vi "Teleop.vi"(10 "Match Info":T2={"Autonomous Elapsed Seconds"=0.0, "TeleOp Elapsed Seconds"=0.0, "Disabled Elapsed Seconds"=0.0, "Visited Autonomous"=FALSE, "Visited TeleOp"=FALSE, "Visited Disabled"=FALSE, "Autonomous Settings"={"Autonomous Style"=enum."Independent", "VI Refnum"=refnum}}, 11 "Call Context":T3) -> ()   [LabVIEW 2020]
doc: "This VI is called for each TeleOp packet received from the DS where the robot is not disabled. It is often used to read from the joysticks and update I/O or to update setpoints for timed control loops. It should complete and return within 20 milliseconds or it may miss DS packets."
uses:
  <vilib>/Rock Robotics/WPI/DriverStation/WPI_DriverStationDerivedRobotMode.ctl
  <vilib>/Rock Robotics/WPI/DriverStation/WPI_DriverStationMatch Info.ctl
  <vilib>/Rock Robotics/WPI/ThirdParty/Phoenix-LabVIEW/Motor Controller/Controls/CTRE_Phoenix_MotorControl_ControlMode.ctl
  <vilib>/Rock Robotics/WPI/ThirdParty/Phoenix-LabVIEW/CANCoder/Get/CTRE_Phoenix_CANcoder_GetSensorData.vi
  <vilib>/Rock Robotics/WPI/ThirdParty/Phoenix-LabVIEW/Pigeon IMU/CTRE_PigeonIMU_GetYPR.vi
panel:
  in  "FR PID gains":T1={"proportional gain (Kc)"=0.01, "integral time (Ti, min)"=0.0, "derivative time (Td, min)"=0.0} {"derivative time (Td, min)" format="%.3f"; "integral time (Ti, min)" format="%.3f"; "proportional gain (Kc)" format="%.6f"}
  in  "FL PID gains":T1={"proportional gain (Kc)"=0.01, "integral time (Ti, min)"=0.0, "derivative time (Td, min)"=0.0} {"derivative time (Td, min)" format="%.3f"; "integral time (Ti, min)" format="%.3f"; "proportional gain (Kc)" format="%.6f"}
  in  "BR PID gains":T1={"proportional gain (Kc)"=0.01, "integral time (Ti, min)"=0.0, "derivative time (Td, min)"=0.0} {"derivative time (Td, min)" format="%.3f"; "integral time (Ti, min)" format="%.3f"; "proportional gain (Kc)" format="%.6f"}
  in  "BL PID gains":T1={"proportional gain (Kc)"=0.01, "integral time (Ti, min)"=0.0, "derivative time (Td, min)"=0.0} {"derivative time (Td, min)" format="%.3f"; "integral time (Ti, min)" format="%.3f"; "proportional gain (Kc)" format="%.6f"}
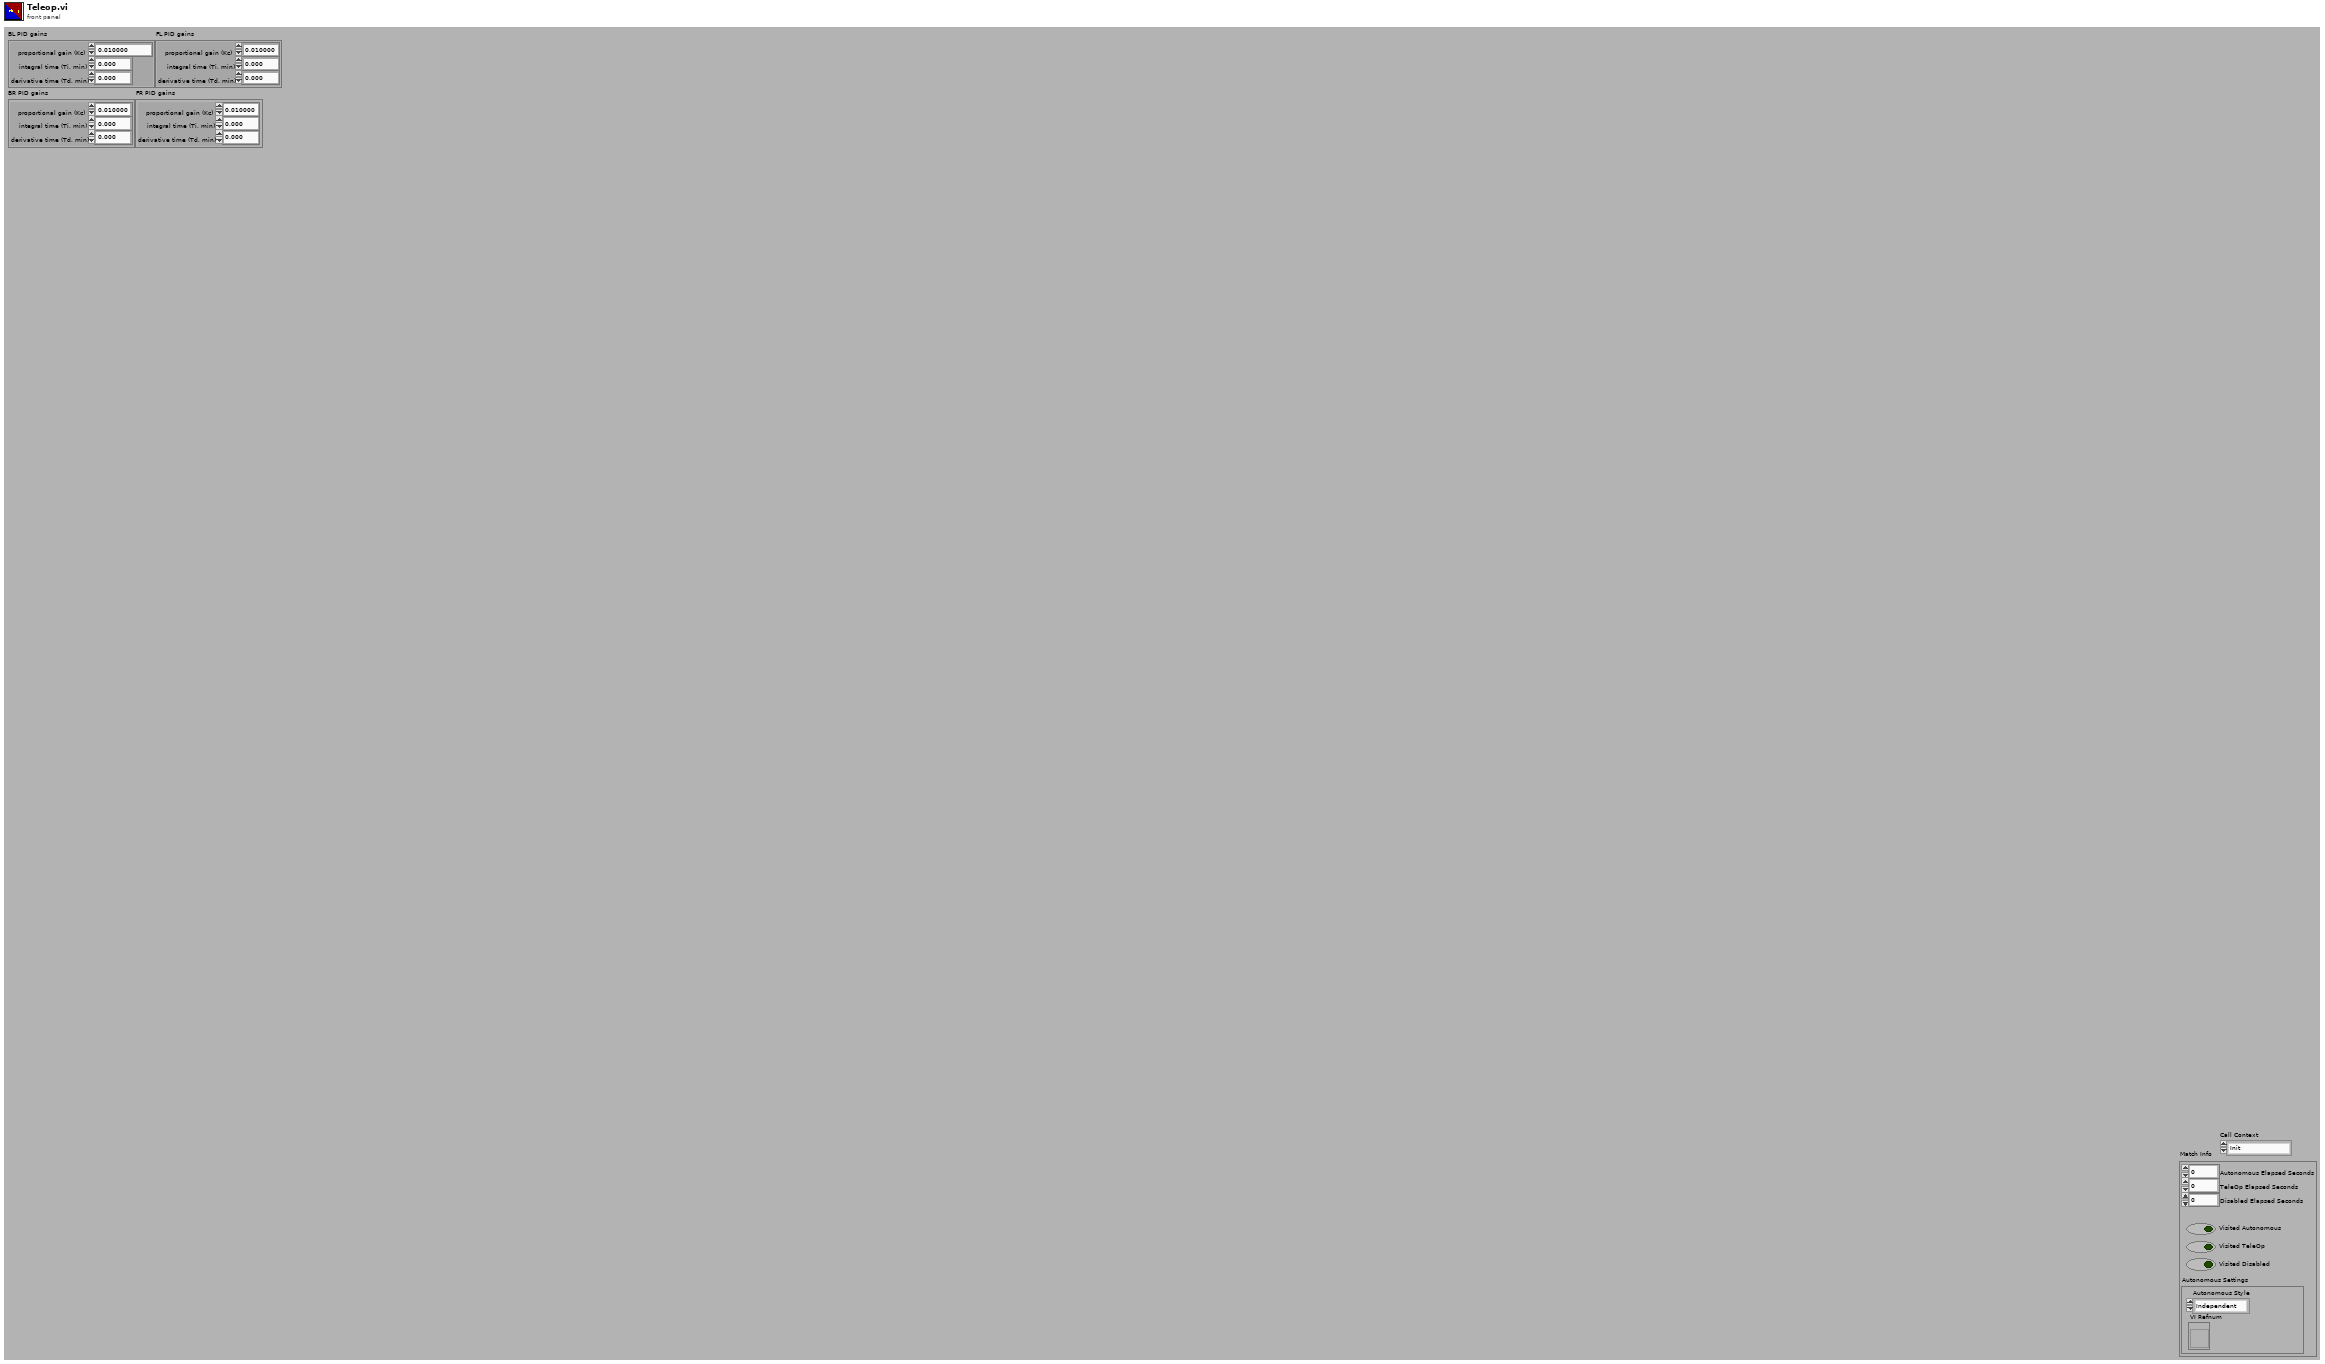
[diagram p1: front panel]
types:
  T1 = cluster{"proportional gain (Kc)":dbl, "integral time (Ti, min)":dbl, "derivative time (Td, min)":dbl}
  T2 = typedef "WPI_DriverStationMatch Info.ctl" = cluster{"Autonomous Elapsed Seconds":dbl, "TeleOp Elapsed Seconds":dbl, "Disabled Elapsed Seconds":dbl, "Visited Autonomous":bool, "Visited TeleOp":bool, "Visited Disabled":bool, "Autonomous Settings":cluster{"Autonomous Style":enum16{"Iterative", "Independent"}, "VI Refnum":refnum<vi>}}
  T3 = typedef "WPI_DriverStationDerivedRobotMode.ctl" = enum16{"Init", "Execute", "Stop"}
  T4 = typedef "CTRE_Phoenix_MotorControl_ControlMode.ctl" = u16
  T5 = cluster{"A":bool, "B":bool, "X":bool, "Y":bool, "Left Bumper":bool, "Right Bumper":bool, "View Button":bool, "Menu Button":bool, "Left Joystick Press":bool, "Right Joystick Press":bool, "Left Thumbpad X Axis":dbl, "Left Thumbpad Y Axis":dbl, "Left Trigger":dbl, "Right Trigger":dbl, "Right Thumbpad X Axis":dbl, "Right Thumbpad Y Axis":dbl, "Driver - Trigger":bool, "Driver - Middle Thumb":bool, "Driver - Left Thumb":bool, "Driver - Right Thumb":bool, "Driver - Left Top Left ":bool, "Driver - Left Top Middle":bool, "Driver - Left Top Right":bool, "Driver - Left Bottom Right":bool, "Driver - Left Bottom Middle":bool, "Driver - Left Bottom Left":bool, "Driver - Right Top Right":bool, "Driver - Right Top Middle":bool, "Driver - Right Top Left":bool, "Driver - Right Bottom Left":bool, "Driver - Right Bottom Middle":bool, "Driver - Right Bottom Right":bool, "Driver - X Axis":dbl, "Driver - Y Axis":dbl, "Driver - Z Axis":dbl}
  T6 = typedef "CTRE_PigeonIMU_DeviceRef.ctl" = cluster{"DeviceStatus":errorcluster, "Device Number":u8, "Type":T7, "Device ID":u32, "Handle":u64, "UsageFrame":u32, "Library Path":path}
  T7 = typedef "CTRE_PigeonIMU_ConnectionType.ctl" = u32
  T8 = typedef "CTRE_Phoenix_CANcoder_DeviceRef.ctl" = cluster{"DeviceStatus":errorcluster, "Device Number":u8, "Handle":u64, "UsageFrame":u32, "Library Path":path}
  T9 = typedef "WPI_MotorControlDeviceRef.ctl" = cluster{"DeviceStatus":errorcluster, "Type":T10, "PWM":cluster{"PWM Channel":T11, "DeadBand":T12}, "CAN":cluster{"Device Number":u8, "SetOutput VI Ref":variant, "GetOutput VI Ref":variant, "Enable VI Ref":variant, "Disable VI Ref":variant, "Data":variant}, "Invert":bool, "DIO PWM":cluster{"PWM \"Enable\" Channel":T11, "DIOChannel":T13, "PWM Rate":dbl}}
  T10 = typedef "WPI_MotorControlType.ctl" = enum16{"PWM", "CAN", "DIO PWM"}
  T11 = typedef "FPGA_DIOPWMChannel.ctl" = enum8{"PWM 0", "PWM 1", "PWM 2", "PWM 3", "PWM 4", "PWM 5", "PWM 6", "PWM 7", "PWM 8", "PWM 9", "PWM MXP 0", "PWM MXP 1", "PWM MXP 2", "PWM MXP 3", "PWM MXP 4", "PWM MXP 5", "PWM MXP 6", "PWM MXP 7", "PWM MXP 8", "PWM MXP 9", "Invalid"}
  T12 = typedef "WPI_PWMDeadband.ctl" = cluster{"Name":string, "maxPositivePwm":i32, "minPositivePwm":i32, "centerPwm":i32, "maxNegativePwm":i32, "minNegativePwm":i32, "angularRange":u16}
  T13 = typedef "FPGA_DIOChannel.ctl" = enum8{"DIO 0", "DIO 1", "DIO 2", "DIO 3", "DIO 4", "DIO 5", "DIO 6", "DIO 7", "DIO 8", "DIO 9", "DIO MXP 0", "DIO MXP 1", "DIO MXP 2", "DIO MXP 3", "DIO MXP 4", "DIO MXP 5", "DIO MXP 6", "DIO MXP 7", "DIO MXP 8", "DIO MXP 9", "DIO MXP 10", "DIO MXP 11", "DIO MXP 12", "DIO MXP 13", "DIO MXP 14", "DIO MXP 15", "SPI Port CS1", "SPI Port CS2", "SPI Port CS3", "SPI Port MISO", "SPI Port MOSI", "Invalid"}
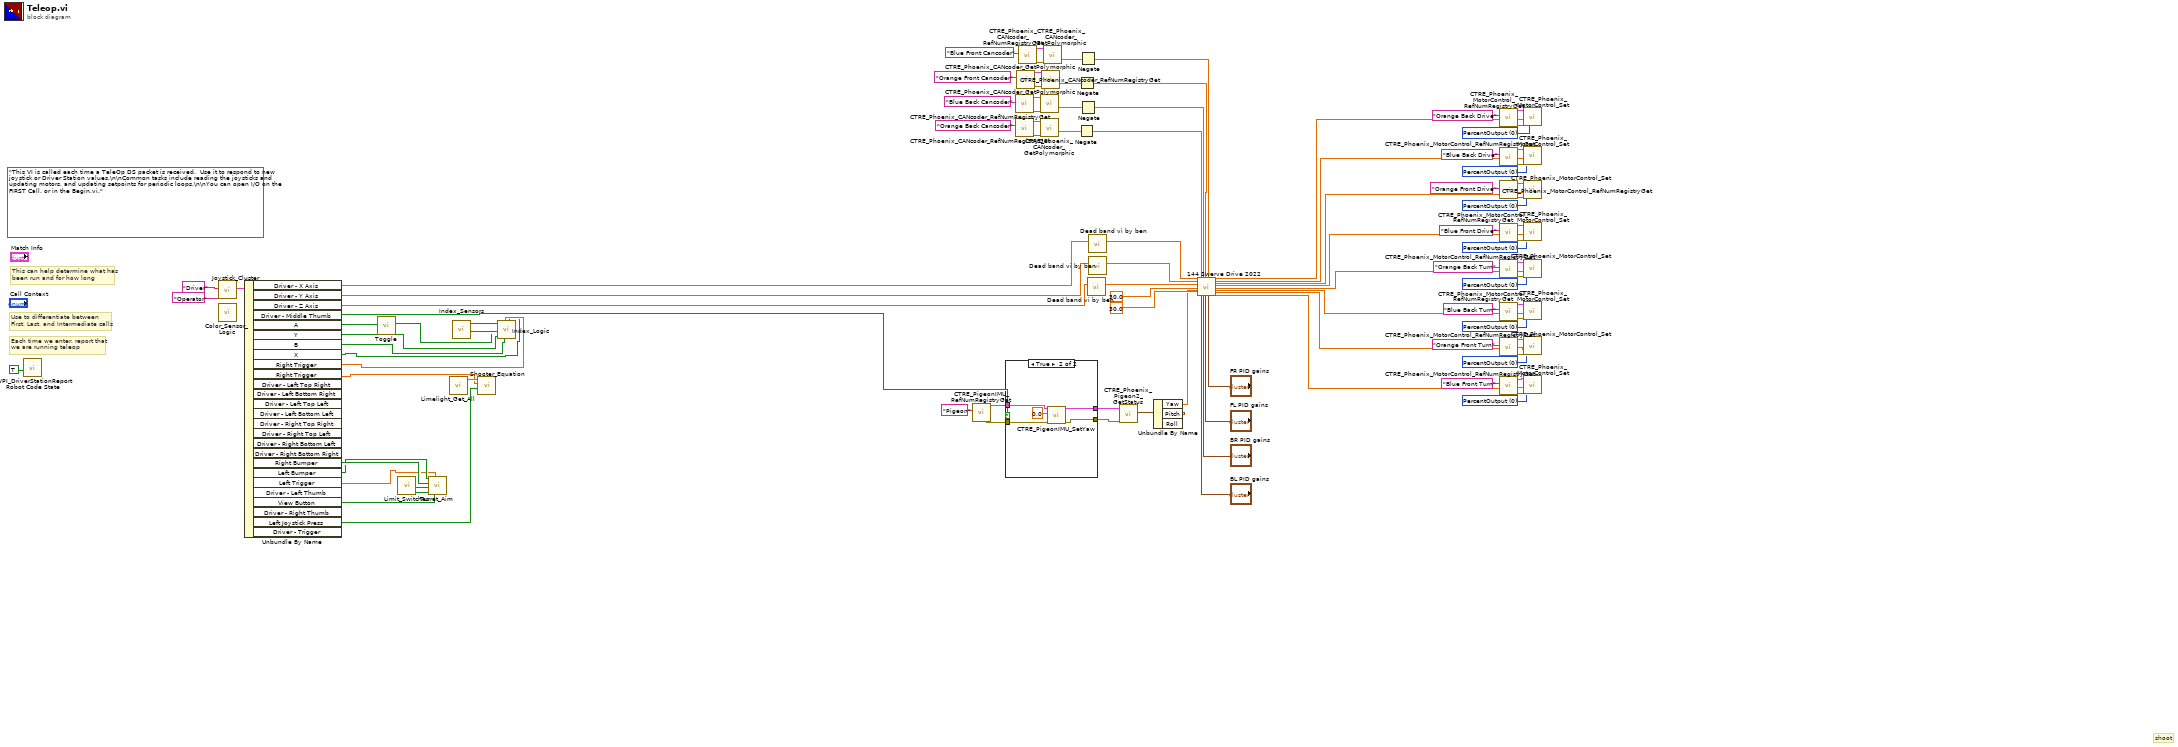
[diagram p0: block diagram]
diagram:
  w14 = T4 0 items=["PercentOutput"=0, "Position"=1, "Velocity"=2, "Current"=3, "Follower"=5, "MotionProfile"=6, "MotionMagic"=7, "MotionProfileArc"=10, "Disabled"=15] ("Control Mode")
  w18 = T4 0 items=["PercentOutput"=0, "Position"=1, "Velocity"=2, "Current"=3, "Follower"=5, "MotionProfile"=6, "MotionMagic"=7, "MotionProfileArc"=10, "Disabled"=15] ("Control Mode")
  w21 = T4 0 items=["PercentOutput"=0, "Position"=1, "Velocity"=2, "Current"=3, "Follower"=5, "MotionProfile"=6, "MotionMagic"=7, "MotionProfileArc"=10, "Disabled"=15] ("Control Mode")
  w25 = T4 0 items=["PercentOutput"=0, "Position"=1, "Velocity"=2, "Current"=3, "Follower"=5, "MotionProfile"=6, "MotionMagic"=7, "MotionProfileArc"=10, "Disabled"=15] ("Control Mode")
  w53 = T4 0 items=["PercentOutput"=0, "Position"=1, "Velocity"=2, "Current"=3, "Follower"=5, "MotionProfile"=6, "MotionMagic"=7, "MotionProfileArc"=10, "Disabled"=15] ("Control Mode")
  w57 = T4 0 items=["PercentOutput"=0, "Position"=1, "Velocity"=2, "Current"=3, "Follower"=5, "MotionProfile"=6, "MotionMagic"=7, "MotionProfileArc"=10, "Disabled"=15] ("Control Mode")
  w60 = T4 0 items=["PercentOutput"=0, "Position"=1, "Velocity"=2, "Current"=3, "Follower"=5, "MotionProfile"=6, "MotionMagic"=7, "MotionProfileArc"=10, "Disabled"=15] ("Control Mode")
  w4 = T4 0 items=["PercentOutput"=0, "Position"=1, "Velocity"=2, "Current"=3, "Follower"=5, "MotionProfile"=6, "MotionMagic"=7, "MotionProfileArc"=10, "Disabled"=15] ("Control Mode")
  (unwired) "This VI is called each time a TeleOp DS packet is received.  Use it to respond to new joystick or Driver Station values.\n\nCommon tasks include reading the joysticks and updating motors, and updating setpoints for periodic loops.\n\nYou can open I/O on the FIRST Call, or in the Begin.vi."
  # "shoot"
  # "Each time we enter, report that\nwe are running teleop"
  # "Use to differentiate between\nFirst, Last, and Intermediate calls"
  # "This can help determine what has\nbeen run and for how long"
  n1 = call <vilib>:"WPI_DriverStationReport Robot Code State.vi"("TeleOp"=TRUE ("Autonomous")) -> ()  [unwired: 10 in, 1 out]
  n2 = call "Joystick_Cluster.vi"("Xbox"="Operator", "Thrustmaster"="Driver") -> ("Joystick Output"=w98:T5)  [unwired: 9 in]
  n3 = call "Color_Sensor_Logic.vi"() -> ()  [unwired: 12 in]
  n4 = Unbundle By Name(w98) -> ("Driver - X Axis"=w36:dbl, "Driver - Y Axis"=w35:dbl, "Driver - Z Axis"=w34:dbl, "Driver - Middle Thumb"=w41:bool, "A"=w92:bool, "Y"=w95:bool, "B"=w94:bool, "X"=w1:bool, "Right Trigger"=w93:dbl, "Right Trigger"=w89:dbl, "Right Bumper"=w86:bool, "Left Bumper"=w85:bool, "Left Trigger"=w84:dbl, "View Button"=w83:bool, "Left Joystick Press"=w2:bool)  [unwired: 11 out]
  n5 = call "Toggle.vi"("Boolean"=w92) -> ("Boolean Out"=w91:bool)
  n6 = call "Limit_Switches.vi"() -> ("Blue Limit Pressed"=w87:bool, "Orange Limit Pressed"=w88:bool)  [unwired: 10 in]
  n7 = call "Turret_Aim.vi"("View Button"=w83, "Left Trigger"=w84, "Orange Limit Pressed"=w88, "Blue Limit Pressed"=w87, "Right Bumper"=w86, "Left Bumper"=w85) -> ()  [unwired: 6 in]
  n8 = call "Limelight_Get_All.vi"() -> ("Ty"=w90:dbl)  [unwired: 10 in, 1 out]
  n9 = call "Index_Sensors.vi"() -> ("Intake Pressed"=w97:bool, "Elevate Pressed"=w96:bool)  [unwired: 9 in, 1 out]
  n10 = call "Shooter_Equation.vi"("Left Bumper"=w2, "Right Trigger"=w89, "Ty"=w90) -> ()  [unwired: 9 in]
  n11 = call "Index_Logic.vi"("Intake Pressed"=w97, "X"=w1, "B"=w94, "Right Trigger"=w93, "Y"=w95, "A"=w91, "Elevate Pressed"=w96) -> ()  [unwired: 5 in]
  n12 = call <vilib>:"CTRE_PigeonIMU_RefNumRegistryGet.vi"("refnum name"="Pigeon") -> ("error out"=w50:errorcluster, "PigeonIMUDevRef"=w51:T6)  [unwired: 9 in]
  n13 = case shown="True" w41 {
    tunnel: w51 -> [w103 w107]
    tunnel: w50 -> [w102 w106]
    tunnel: [w102 w105] -> w49
    tunnel: [w103 w104] -> w48
    frame False {
    }
    frame True {
      n14 = call <vilib>:"CTRE_PigeonIMU_SetYaw.vi"("error in (no error)"=w106, "Value"=0.0, "PigeonIMUDevRef"=w107) -> ("error out"=w105:errorcluster, "PigeonIMUDevRef"=w104:T6)  [unwired: 7 in]
    }
  }
  n15 = call <vilib>:"CTRE_Phoenix_CANcoder_RefNumRegistryGet.vi"("refnum name"="Blue Back Cancoder") -> ("error out"=w77:errorcluster, "CTRE_CANcoder_DeviceRef"=w78:T8)  [unwired: 9 in]
  n16 = call <vilib>:"CTRE_Phoenix_CANcoder_RefNumRegistryGet.vi"("refnum name"="Orange Back Cancoder") -> ("error out"=w79:errorcluster, "CTRE_CANcoder_DeviceRef"=w80:T8)  [unwired: 9 in]
  n17 = call <vilib>:"CTRE_Phoenix_CANcoder_RefNumRegistryGet.vi"("refnum name"="Orange Front Cancoder") -> ("error out"=w81:errorcluster, "CTRE_CANcoder_DeviceRef"=w82:T8)  [unwired: 9 in]
  n18 = call <vilib>:"CTRE_Phoenix_CANcoder_RefNumRegistryGet.vi"("refnum name"="Blue Front Cancoder") -> ("error out"=w75:errorcluster, "CTRE_CANcoder_DeviceRef"=w76:T8)  [unwired: 9 in]
  n19 = call-poly <vilib>:"CTRE_Phoenix_CANcoder_GetPolymorphic.vi"("CTRE_CANcoder_DeviceRef"=w78, "error in"=w77) -> ("Absolute Position"=w70:dbl)  [unwired: 9 in, 4 out]
  n20 = call-poly <vilib>:"CTRE_Phoenix_CANcoder_GetPolymorphic.vi"("CTRE_CANcoder_DeviceRef"=w80, "error in"=w79) -> ("Absolute Position"=w68:dbl)  [unwired: 9 in, 4 out]
  n21 = call-poly <vilib>:"CTRE_Phoenix_CANcoder_GetPolymorphic.vi"("CTRE_CANcoder_DeviceRef"=w82, "error in"=w81) -> ("Absolute Position"=w67:dbl)  [unwired: 9 in, 4 out]
  n22 = call-poly <vilib>:"CTRE_Phoenix_CANcoder_GetPolymorphic.vi"("CTRE_CANcoder_DeviceRef"=w76, "error in"=w75) -> ("Absolute Position"=w69:dbl)  [unwired: 9 in, 4 out]
  n23 = Negate(x=w68) -> (-x=w40:dbl)
  n24 = Negate(x=w67) -> (-x=w38:dbl)
  n25 = Negate(x=w69) -> (-x=w37:dbl)
  n26 = Negate(x=w70) -> (-x=w39:dbl)
  n27 = call "Dead band vi by ben.vi"("Numeric"=w34) -> ("Deadbanded Value"=w31:dbl)  [unwired: 10 in]
  n28 = call "Dead band vi by ben.vi"("Numeric"=w36) -> ("Deadbanded Value"=w33:dbl)  [unwired: 10 in]
  n29 = call "Dead band vi by ben.vi"("Numeric"=w35) -> ("Deadbanded Value"=w32:dbl)  [unwired: 10 in]
  n30 = call-poly <vilib>:"CTRE_Phoenix_Pigeon2_GetStatus.vi"("error in (no error)"=w49, "PigeonIMUDevRef"=w48) -> ("Yaw Pitch Roll"=w46:cluster{"Yaw":dbl, "Pitch":dbl, "Roll":dbl})  [unwired: 7 in, 2 out]
  n31 = Unbundle By Name(w46) -> ("Yaw"=w3:dbl)  [unwired: 2 out]
  n32 = call "144 Swerve Drive 2022.vi"("Joystick X"=w33, "Joystick Y"=w32, "Joystick Z"=w31, "Robot Length(in.)"=30.0, "Robot Width(in.)"=30.0, "Gyro"=w3, "BL_Steer_Encoder"=w40, "BL PID gains"="BL PID gains", "BR_Steer_Encoder"=w39, "BR PID gains"="BR PID gains", "FL_Steer_Encoder"=w38, "FL PID gains"="FL PID gains", "FR_Steer_Encoder"=w37, "FR PID gains"="FR PID gains") -> ("Throttle BL"=w12:dbl, "Throttle BR"=w11:dbl, "Throttle FL"=w10:dbl, "Throttle FR"=w9:dbl, "BL_STEER_MOTOR_OUTPUT"=w8:dbl, "BR_STEER_MOTOR_OUTPUT"=w7:dbl, "FL_STEER_MOTOR_OUTPUT"=w6:dbl, "FR_STEER_MOTOR_OUTPUT"=w5:dbl)  [unwired: 6 in]
  n33 = call <vilib>:"CTRE_Phoenix_MotorControl_RefNumRegistryGet.vi"("refnum name"="Orange Back Drive") -> ("error out"=w65:errorcluster, "PhoenixMotorControlDevRef"=w66:T9)  [unwired: 9 in]
  n34 = call <vilib>:"CTRE_Phoenix_MotorControl_RefNumRegistryGet.vi"("refnum name"="Blue Back Drive") -> ("error out"=w62:errorcluster, "PhoenixMotorControlDevRef"=w63:T9)  [unwired: 9 in]
  n35 = call <vilib>:"CTRE_Phoenix_MotorControl_RefNumRegistryGet.vi"("refnum name"="Orange Front Drive") -> ("error out"=w59:errorcluster, "PhoenixMotorControlDevRef"=w56:T9)  [unwired: 9 in]
  n36 = call <vilib>:"CTRE_Phoenix_MotorControl_RefNumRegistryGet.vi"("refnum name"="Blue Front Drive") -> ("error out"=w55:errorcluster, "PhoenixMotorControlDevRef"=w52:T9)  [unwired: 9 in]
  n37 = call <vilib>:"CTRE_Phoenix_MotorControl_RefNumRegistryGet.vi"("refnum name"="Orange Back Turn") -> ("error out"=w27:errorcluster, "PhoenixMotorControlDevRef"=w28:T9)  [unwired: 9 in]
  n38 = call <vilib>:"CTRE_Phoenix_MotorControl_RefNumRegistryGet.vi"("refnum name"="Blue Back Turn") -> ("error out"=w23:errorcluster, "PhoenixMotorControlDevRef"=w24:T9)  [unwired: 9 in]
  n39 = call <vilib>:"CTRE_Phoenix_MotorControl_RefNumRegistryGet.vi"("refnum name"="Orange Front Turn") -> ("error out"=w20:errorcluster, "PhoenixMotorControlDevRef"=w17:T9)  [unwired: 9 in]
  n40 = call <vilib>:"CTRE_Phoenix_MotorControl_RefNumRegistryGet.vi"("refnum name"="Blue Front Turn") -> ("error out"=w16:errorcluster, "PhoenixMotorControlDevRef"=w13:T9)  [unwired: 9 in]
  n41 = call <vilib>:"CTRE_Phoenix_MotorControl_Set.vi"("error in (no error)"=w65, "Output"=w12, "Control Mode"=w4, "PhoenixMotorControlDevRef"=w66) -> ()  [unwired: 6 in, 2 out]
  n42 = call <vilib>:"CTRE_Phoenix_MotorControl_Set.vi"("error in (no error)"=w62, "Output"=w11, "Control Mode"=w60, "PhoenixMotorControlDevRef"=w63) -> ()  [unwired: 6 in, 2 out]
  n43 = call <vilib>:"CTRE_Phoenix_MotorControl_Set.vi"("error in (no error)"=w59, "Output"=w10, "Control Mode"=w57, "PhoenixMotorControlDevRef"=w56) -> ()  [unwired: 6 in, 2 out]
  n44 = call <vilib>:"CTRE_Phoenix_MotorControl_Set.vi"("error in (no error)"=w55, "Output"=w9, "Control Mode"=w53, "PhoenixMotorControlDevRef"=w52) -> ()  [unwired: 6 in, 2 out]
  n45 = call <vilib>:"CTRE_Phoenix_MotorControl_Set.vi"("error in (no error)"=w27, "Output"=w8, "Control Mode"=w25, "PhoenixMotorControlDevRef"=w28) -> ()  [unwired: 6 in, 2 out]
  n46 = call <vilib>:"CTRE_Phoenix_MotorControl_Set.vi"("error in (no error)"=w23, "Output"=w7, "Control Mode"=w21, "PhoenixMotorControlDevRef"=w24) -> ()  [unwired: 6 in, 2 out]
  n47 = call <vilib>:"CTRE_Phoenix_MotorControl_Set.vi"("error in (no error)"=w20, "Output"=w6, "Control Mode"=w18, "PhoenixMotorControlDevRef"=w17) -> ()  [unwired: 6 in, 2 out]
  n48 = call <vilib>:"CTRE_Phoenix_MotorControl_Set.vi"("error in (no error)"=w16, "Output"=w5, "Control Mode"=w14, "PhoenixMotorControlDevRef"=w13) -> ()  [unwired: 6 in, 2 out]
